vi "WPI_CameraGet Enum Sensor Property.vi"(8 "error in (no error)":errorcluster, 9 "Strings":string[](array[string]), 10 "Property Name":string, 11 "CameraDevRef":T1) -> (0 "error out":errorcluster, 2 "Enum Int Value":i32, 3 "CameraDevRef out":T1)   [LabVIEW 2017]
doc: "This software is licensed. Open the labview\\readme\\WPI Robotics Library Open Source License.txt file for more information."
uses:
  <vilib>/Rock Robotics/WPI/Camera/WPI_CameraDevRef.ctl
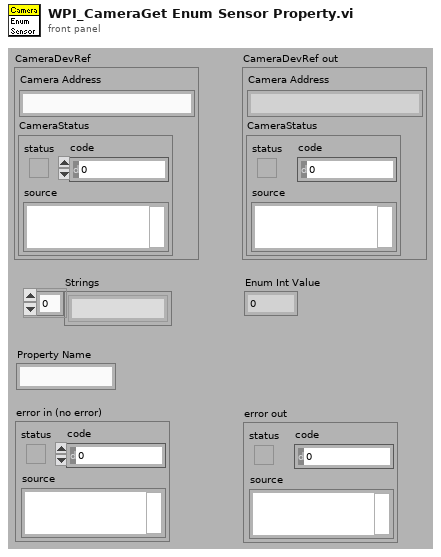
[diagram p1: front panel]
types:
  T1 = typedef "WPI_CameraDevRef.ctl" = cluster{"Camera Address":string, "CameraStatus":errorcluster}
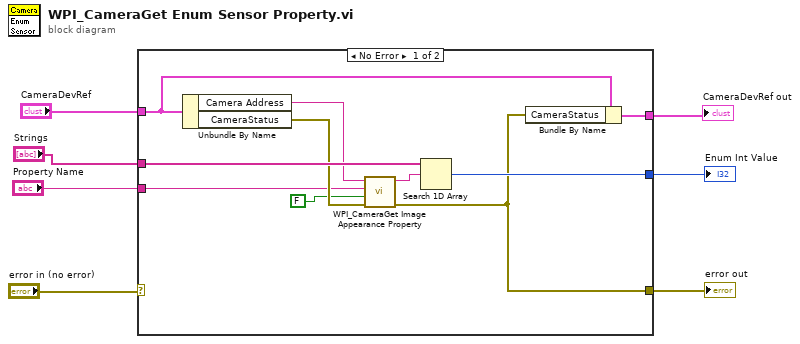
[diagram p0: block diagram]
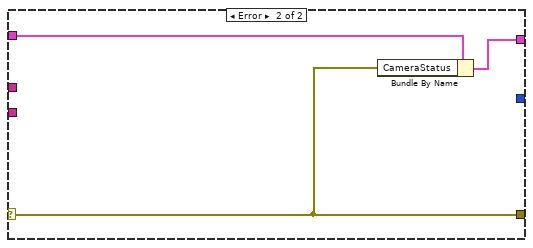
[diagram p2: hidden frame]
diagram:
  n1 = case shown="No Error" "error in (no error)" {
    selector: "error in (no error)" -> [_ w18]
    tunnel: [w17 w19] -> w7
    tunnel: [w12 w18] -> w6
    tunnel: "CameraDevRef" -> [w16 w20]
    tunnel: "Property Name" -> [w9 _]
    tunnel: [w15 _] -> w3
    tunnel: "Strings" -> [w14 _]
    frame No Error {
      n2 = Unbundle By Name(w16) -> ("Camera Address"=w10:string, "CameraStatus"=w11:errorcluster)
      n3 = call <vilib>:"WPI_CameraGet Image Appearance Property.vi"("error in (no error)"=w11, "Appearance"=FALSE, "Prop String"=w9, "address"=w10) -> ("error out"=w12:errorcluster, "Value"=w13:string)  [unwired: 6 in]
      n4 = Search 1D Array(1D array=w14, element=w13) -> (index of element=w15:i32)  [unwired: 1 out]
      n5 = Bundle By Name(cluster=w16, "CameraStatus"=w12) -> (w17:T1)
    }
    frame Error {
      n6 = Bundle By Name(cluster=w20, "CameraStatus"=w18) -> (w19:T1)
    }
  }
  "CameraDevRef out" <- w7
  "error out" <- w6
  "Enum Int Value" <- w3
